vi "FTW-Actor-Publisher-Add.vi"(0 "FTW-ActorInstance In":refnum<class "FTW-ActorInstance.lvclass">, 5 "Publisher Name":string, 7 "Publisher URI":string, 11 "error in":errorcluster, 12 "Send Buffer Depth (1)":i32=1, 13 "Send Timeout (-1)":i32=-1) -> (4 "FTW-ActorInstance Out":refnum<class "FTW-ActorInstance.lvclass">, 15 "error out":errorcluster)   [LabVIEW 2015, in "FTW-ActorInstance.lvclass"]
uses:
  FTW-ActorInstance.lvclass
  FTW-ActorInstance.lvclass/FTW-ActorInstance.ctl
  Publisher/FTW-Publisher.lvclass
  Ether/FTW-Ether.lvclass
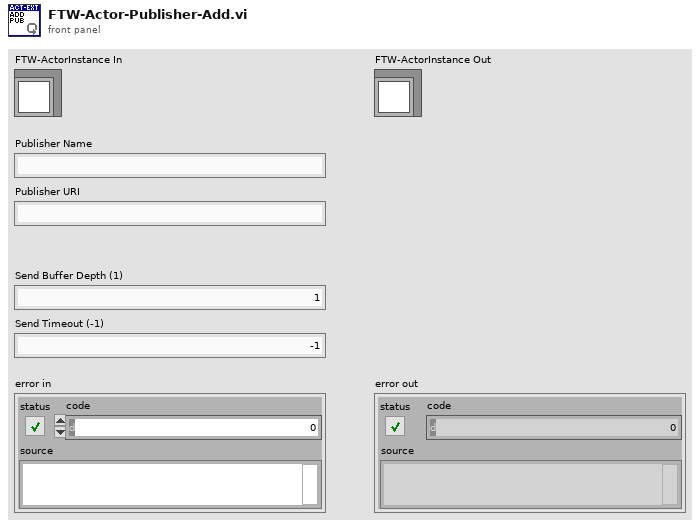
[diagram p1: front panel]
types:
  T1 = cluster{"Name":string, "URI":string, "Publisher":refnum<class "FTW-Publisher.lvclass">}[]
  T2 = cluster{"Publisher Name":string, "Actual Address":string, "FTW-Publisher Out":refnum<class "FTW-Publisher.lvclass">}
  T3 = cluster{"Publisher Name":string, "Actual Address":string, "FTW-Publisher Out":refnum<class "FTW-Publisher.lvclass">}[]
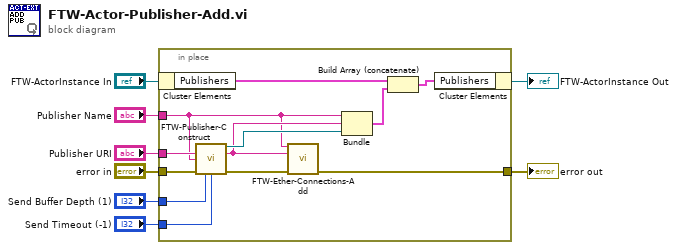
[diagram p0: block diagram]
diagram:
  n1 = in-place {
    in-place-border: "Publisher URI" -> [w20]
    in-place-border: "Publisher Name" -> [w9]
    in-place-border: "Send Buffer Depth (1)" -> [w15]
    in-place-border: "Send Timeout (-1)" -> [w14]
    in-place-border: [w11] -> w2
    in-place-border: "error in" -> [w12]
    n2 = in-place-cluster #1("FTW-ActorInstance In") -> ("Publishers"=w17:T1)
    n3 = call "FTW-Publisher-Construct.vi"("Address"=w20, "Identity"=w9, "error in"=w12, "Send Buffer Depth (1)"=w15, "Send Timeout (-1)"=w14) -> ("FTW-Publisher Out"=w16:refnum<class "FTW-Publisher.lvclass">, "Actual Address"=w10:string, "error out"=w13:errorcluster)  [unwired: 8 in]
    n4 = call "FTW-Ether-Connections-Add.vi"("Connection"=w9, "Address"=w10, "error in"=w13) -> ("error out"=w11:errorcluster)  [unwired: 12 in]
    n5 = Bundle("Publisher Name"=w9, "Actual Address"=w10, "FTW-Publisher Out"=w16) -> (w19:T2)  [unwired: 1 in]
    n6 = Build Array (concatenate)(w17, w19) -> (w18:T3)
    n7 = in-place-cluster #1("Publishers"=w18) -> (→"FTW-ActorInstance Out":refnum<class "FTW-ActorInstance.lvclass">)
  }
  "error out" <- w2
